vi "PAQmem_Read Size.vi"(8 "error in (no error)":errorcluster, 11 "PAQ-memory in":refnum<class "PAQ-memory.lvclass">) -> (0 "error out":errorcluster, 2 "Size":i32, 3 "PAQ-memory out":refnum<class "PAQ-memory.lvclass">)   [LabVIEW 2014, in "PAQ-memory.lvclass"]
uses:
  PAQ-memory.lvclass
  PAQ-memory.lvclass/PAQ-memory.ctl
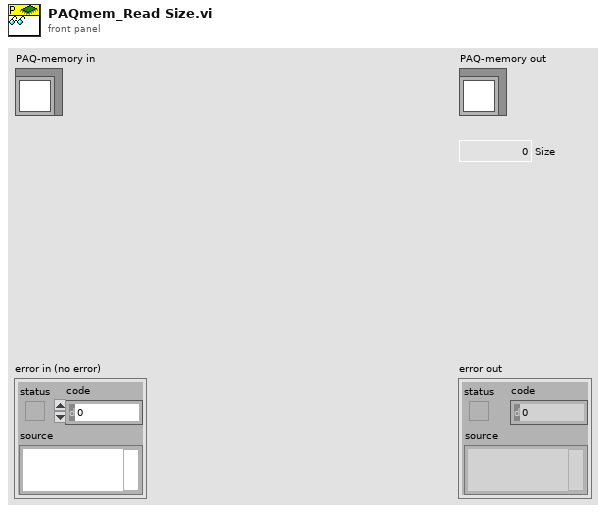
[diagram p1: front panel]
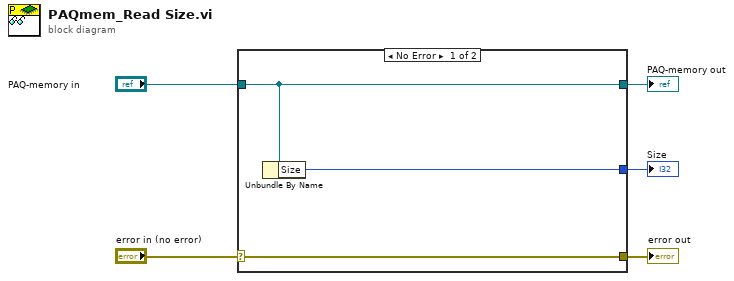
[diagram p0: block diagram]
diagram:
  n1 = case shown="No Error" "error in (no error)" {
    selector: "error in (no error)" -> [w8 w9]
    tunnel: [w8 w9] -> w4
    tunnel: [w7 w10] -> w2
    tunnel: "PAQ-memory in" -> [w7 w10]
    tunnel: [w6 _] -> w1
    frame No Error {
      n2 = Unbundle By Name(w7) -> ("Size"=w6:i32)
    }
    frame Error {
    }
  }
  "error out" <- w4
  "PAQ-memory out" <- w2
  "Size" <- w1
